vi "Visa_Write read_UI SETPIN.vi"(0 "Cypress in":refnum<class "Cypress.lvclass">, 1 "VISA Refnum in":refnum<visa-resource-name>, 3 "Command to Send":string, 5 "error in (no error)":errorcluster) -> (14 "Cypress out":refnum<class "Cypress.lvclass">, 15 "VISA Refnum out":refnum<visa-resource-name>, 16 "Puerto":string, 17 "Valor Pin":string, 18 "Pin":bool, 19 "error out":errorcluster)   [LabVIEW 2020, in "Cypress.lvclass"]
uses:
  Cypress.lvclass
  Abstract/Serial Device/Combo Box Devices.ctl
  Abstract/Serial Device/Combo Box Comandos.ctl
  UI Actor/UI Actor.lvclass
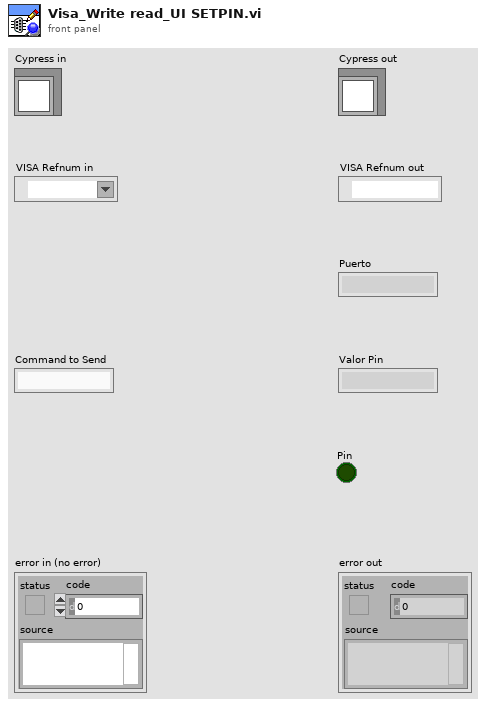
[diagram p1: front panel]
types:
  T1 = typedef "Combo Box Comandos.ctl" = string
  T2 = typedef "Combo Box Devices.ctl" = string
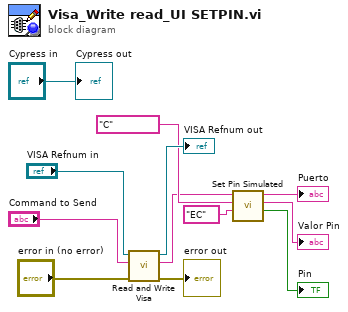
[diagram p0: block diagram]
diagram:
  n1 = call "Read and Write Visa.vi"("error in (no error)"="error in (no error)", "Command to Send"="Command to Send", "VISA Refnum in"="VISA Refnum in") -> ("error out"=→"error out":errorcluster, "Expected Response out"=w2:string, "VISA Refnum out"=→"VISA Refnum out":refnum<visa-resource-name>)  [unwired: 6 in]
  n2 = call "Set Pin Simulated.vi"("Command"=T1 "EC", "Serial Devide Brand"=T2 "C", "Command to Send"=w2) -> ("Pin"=→"Pin":bool, "Valor Pin"=→"Valor Pin":string, "Puerto"=→"Puerto":string)  [unwired: 6 in]
  "Cypress out" <- "Cypress in"
